vi "AssertVIFPStateClosed.vi"(0 "VI Reference In":refnum<vi>, 1 "Label":string, 2 "Assert Only? (F)":bool, 11 "Error In":errorcluster, 12 "Assert Interval(10 ms)":u32=10, 13 "Timeout(5 sec)":dbl=5.0) -> (4 "VI Reference Out":refnum<vi>, 6 "Asserted Value":T1(ring), 15 "Error Out":errorcluster)   [LabVIEW 2016, in "Drona.lvlib" / "AssertVI.lvlib"]
doc: "Asserts if the Front panel of the VI is in Closed state.\nThe input control name is given as a string , incase of path, use delimiters inbetween the path."
uses:
  AssertVI.lvlib
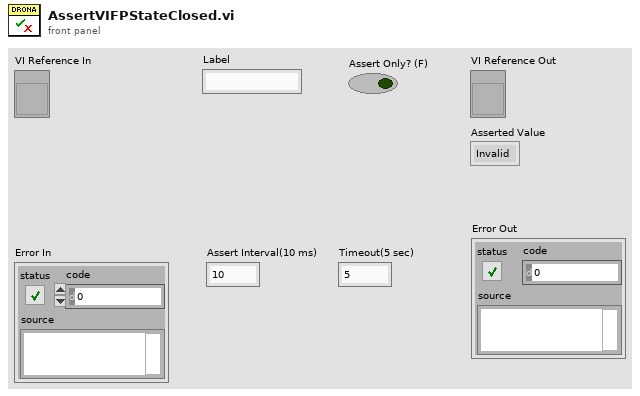
[diagram p1: front panel]
types:
  T1 = enum32{"Invalid", "Standard", "Closed", "Hidden", "Minimized", "Maximized"}
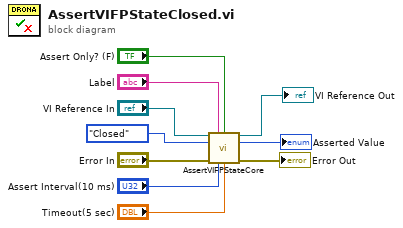
[diagram p0: block diagram]
diagram:
  n1 = call "AssertVIFPStateCore.vi"("VI Reference In"="VI Reference In", "Label"="Label", "Assert Only? (F)"="Assert Only? (F)", "FP State"=T1."Closed", "Error In"="Error In", "Assert Interval(10 ms)"="Assert Interval(10 ms)", "Timeout(5 sec)"="Timeout(5 sec)") -> ("VI Reference Out"=→"VI Reference Out":refnum<vi>, "Asserted Value"=→"Asserted Value":T1, "Error Out"=→"Error Out":errorcluster)  [unwired: 6 in]
